vi "MergeFileConfig.vi"(4 "error in (no error)":errorcluster, 7 "ProjetIN":string) -> (0 "error out":errorcluster, 2 "MergeFileConfigOUT":T1, 3 "ProjetOUT":string)   [LabVIEW 2017]
uses:
  DefDeType/WhichPath.ctl
  DefDeType/MergeFileConfig.ctl
panel:
  out "Nortek File exists":bool
  out "Hexapod file exists":bool
  out "Qualisys File exists":bool
  out "Valise Waveforms":waveform(dbl)[](graph)
  in  "Cancel":bool
  in  "Ok":bool
  in  "MergeFileConfig":T1
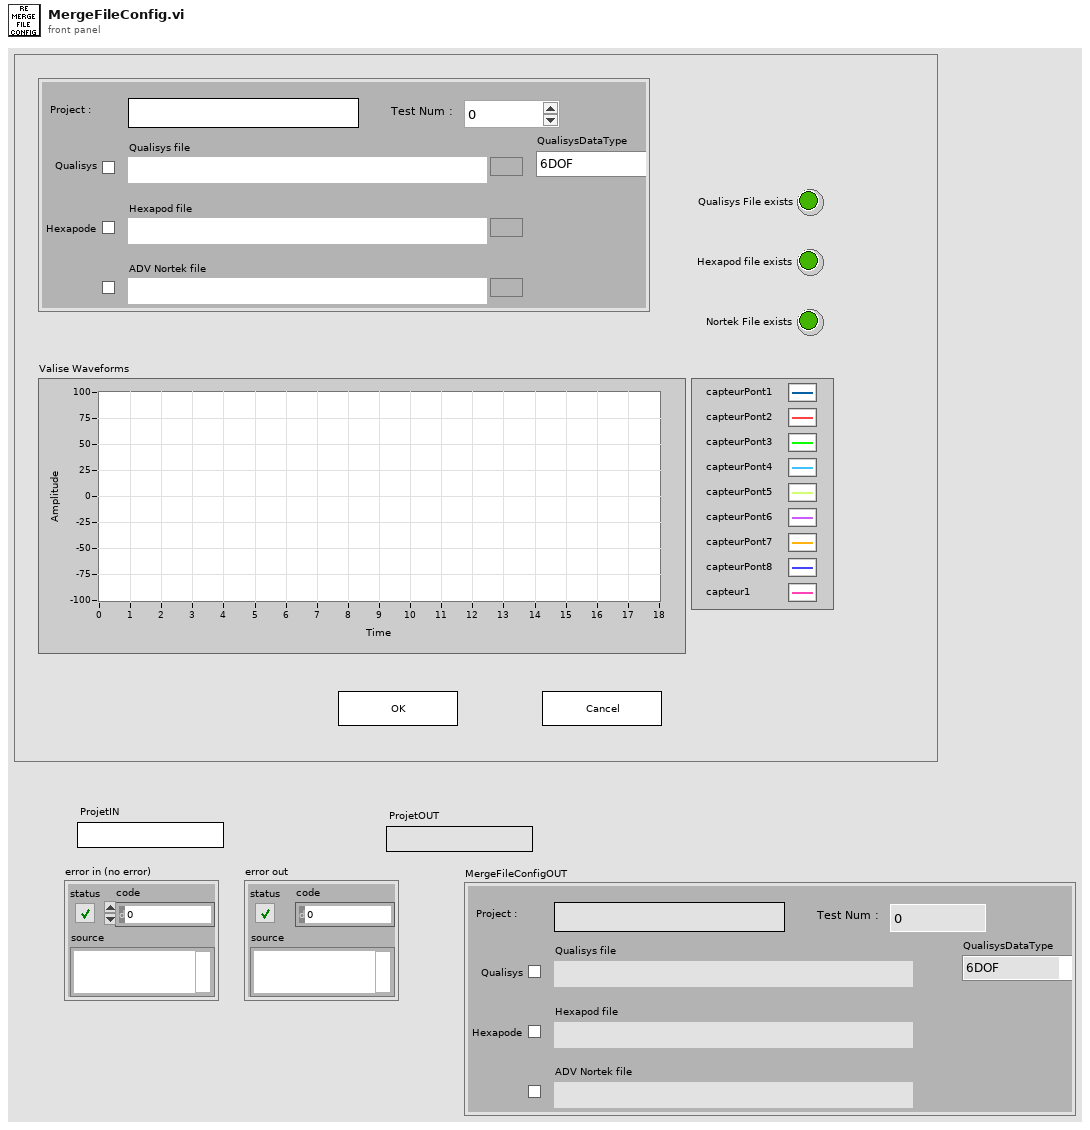
[diagram p1: front panel]
types:
  T1 = typedef "MergeFileConfig.ctl" = cluster{"Test Num : ":u32, "Project :":string, "Qualisys file":path, "Hexapod file":path, "ADV Nortek file":path, "QualisysDataType":enum16{"6DOF", "3DTracking", "6DOF + 3D"}, "Qualisys":bool, "Hexapode":bool, "ADV Nortek":bool}
  T2 = typedef "WhichPath.ctl" = enum16{"DossierProjet", "Config", "Meas", "MeasPCI", "MeasCRIO1", "MeasCRIO2", "MeasQualisys", "MeasHBM", "MeasTDMS", "Fig", "Res"}
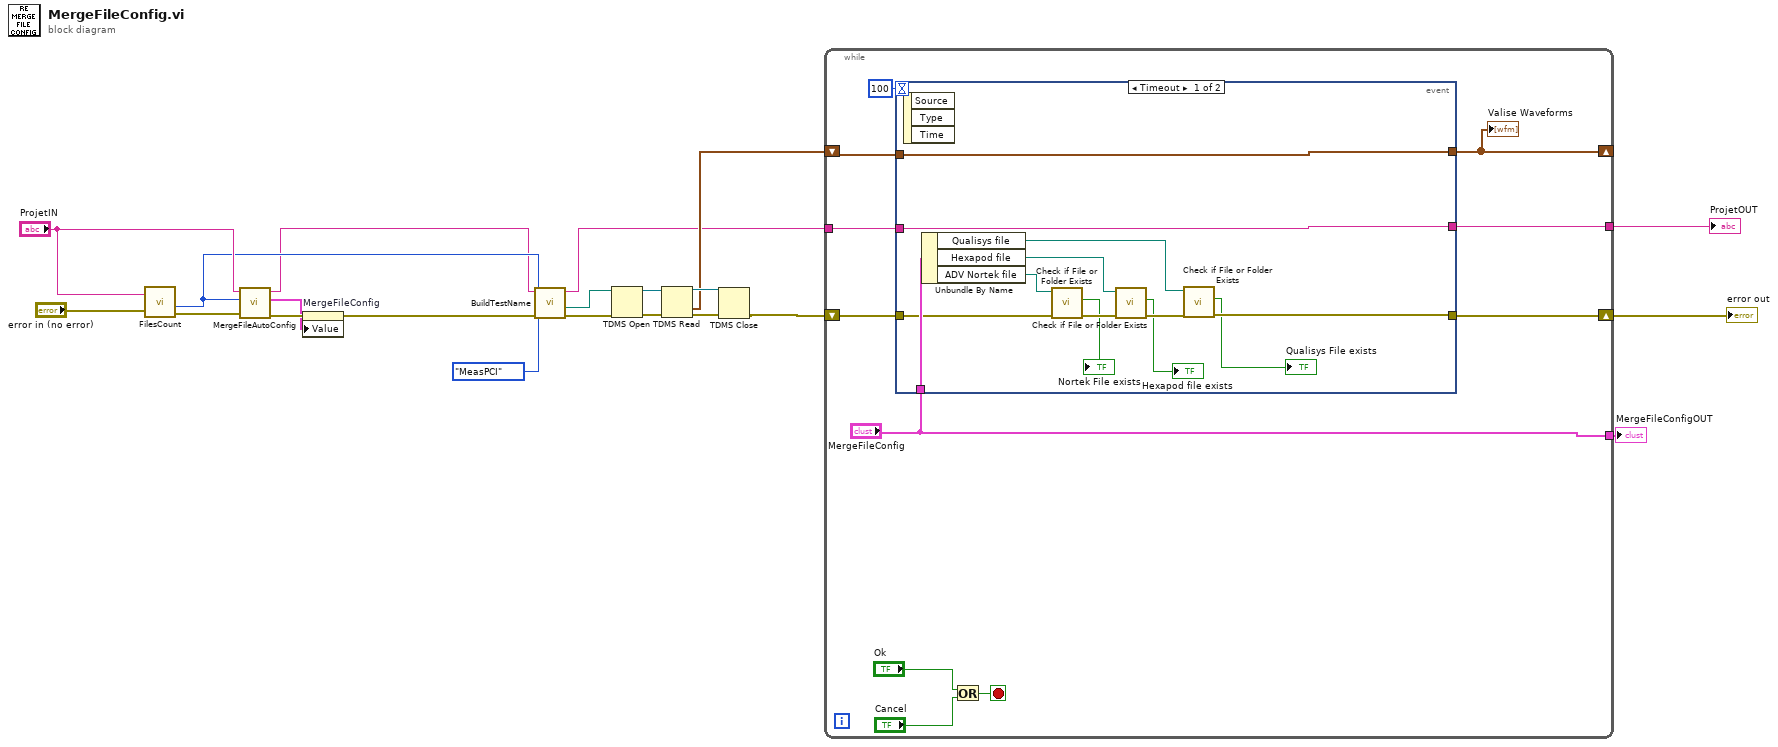
[diagram p0: block diagram]
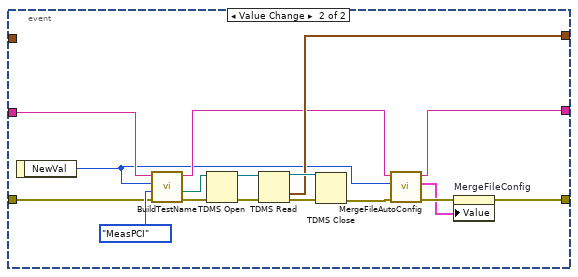
[diagram p2: hidden frame]
diagram:
  n1 = call "FilesCount.vi"("NomProjet"="ProjetIN", "entrée d'erreur"="error in (no error)") -> ("NextTestNum"=w10:u32, "sortie d'erreur"=w20:errorcluster)  [unwired: 4 out]
  n2 = call "MergeFileAutoConfig.vi"("error in (no error)"=w20, "test num"=w10, "ProjetIN"="ProjetIN") -> ("error out"=w19:errorcluster, "MergeFileConfigOUT"=w1:T1, "ProjetOUT"=w2:string)  [unwired: 2 in]
  n3 = property on="MergeFileConfig" class="Clust (strict)"(error in=w19, "Value"=w1) -> (error out=w12:errorcluster)  [unwired: 1 in, 1 out]
  n4 = call "BuildTestName.vi"("entrée d'erreur"=w12, "WhichPath?"=WhichPath."MeasPCI", "NextTestNum"=w10, "NomProjet"=w2) -> ("sortie d'erreur"=w14:errorcluster, "cheminProchainFichier"=w13:path, "NomProjetOut"=w6:string)  [unwired: 1 in, 1 out]
  n5 = TDMS Open(8:w14, 11:w13) -> (0:w17:errorcluster, 3:w18:refnum<k34>)  [unwired: 5 in]
  n6 = TDMS Read(0:w18, 11:w17) -> (4:w16:refnum<k34>, 10:w7:waveform(dbl)[], 15:w15:errorcluster)  [unwired: 6 in, 3 out]
  n7 = TDMS Close(8:w15, 11:w16) -> (0:w8:errorcluster)  [unwired: 1 out]
  n8 = while {
    shift-right: [w23] -> w4
    shift-left: w8 -> [w29]
    shift-right: [w27] -> _
    shift-left: w7 -> [w28]
    tunnel: w6 -> [w26]
    tunnel: [w25] -> w5
    tunnel: ["MergeFileConfig"] -> w3
    stop <- w31 stop-if-true
    n9 = event shown="[0] Timeout" {
      selector: _ -> [_ _]
      dyn-events: _ -> [_ _]
      timeout: 100 ("millisecond multiple") -> [_ _]
      tunnel: w29 -> [w42 w61]
      tunnel: [w36 w50] -> w23
      tunnel: w28 -> [w45 _]
      tunnel: [w45 w54] -> w27
      tunnel: w26 -> [w44 w53]
      tunnel: [w44 w46] -> w25
      tunnel: "MergeFileConfig" -> [w43 _]
      event Timeout {
        n10 = event-data() -> ()  [unwired: 1 in, 3 out]
        n11 = Unbundle By Name(w43) -> ("Qualisys file"=w37:path, "Hexapod file"=w38:path, "ADV Nortek file"=w39:path)
        n12 = call <vilib>:"Check if File or Folder Exists.vi"("error in (no error)"=w42, "path"=w39) -> ("error out"=w41:errorcluster, "file or folder exists?"=→"Nortek File exists":bool)  [unwired: 7 in, 1 out]
        n13 = call <vilib>:"Check if File or Folder Exists.vi"("error in (no error)"=w41, "path"=w38) -> ("error out"=w40:errorcluster, "file or folder exists?"=→"Hexapod file exists":bool)  [unwired: 7 in, 1 out]
        n14 = call <vilib>:"Check if File or Folder Exists.vi"("error in (no error)"=w40, "path"=w37) -> ("error out"=w36:errorcluster, "file or folder exists?"=→"Qualisys File exists":bool)  [unwired: 7 in, 1 out]
      }
      event Value Change {
        n15 = event-data() -> ("NewVal"=w48:u32)  [unwired: 1 in]
        n16 = call "BuildTestName.vi"("entrée d'erreur"=w61, "WhichPath?"=WhichPath."MeasPCI", "NextTestNum"=w48, "NomProjet"=w53) -> ("sortie d'erreur"=w60:errorcluster, "cheminProchainFichier"=w56:path, "NomProjetOut"=w49:string)  [unwired: 1 in, 1 out]
        n17 = TDMS Open(8:w60, 11:w56) -> (0:w57:errorcluster, 3:w55:refnum<k34>)  [unwired: 5 in]
        n18 = TDMS Read(0:w55, 11:w57) -> (4:w58:refnum<k34>, 10:w54:waveform(dbl)[], 15:w59:errorcluster)  [unwired: 6 in, 3 out]
        n19 = TDMS Close(8:w59, 11:w58) -> (0:w51:errorcluster)  [unwired: 1 out]
        n20 = call "MergeFileAutoConfig.vi"("error in (no error)"=w51, "test num"=w48, "ProjetIN"=w49) -> ("error out"=w52:errorcluster, "MergeFileConfigOUT"=w47:T1, "ProjetOUT"=w46:string)  [unwired: 2 in]
        n21 = property on="MergeFileConfig" class="Clust (strict)"(error in=w52, "Value"=w47) -> (error out=w50:errorcluster)  [unwired: 1 in, 1 out]
      }
    }
    "Valise Waveforms" <- w27
    n22 = Or(x="Ok", y="Cancel") -> (x .or. y?=w31:bool)
  }
  "ProjetOUT" <- w5
  "error out" <- w4
  "MergeFileConfigOUT" <- w3
